vi "CheckModuleID.vi"(8 "Error In":errorcluster, 11 "Modle ID Array In":string[][](array[string])=[["12E", "4E"]]) -> (0 "Error Out":errorcluster, 3 "Modle ID ArrayOut":string[][](array[string])=[["12E", "4E"]])   [LabVIEW 2018, in "SensorPlugins.lvlib" / "RoomAlert.lvclass"]
doc: "Checks the Module ID to ensure we are only sending commands to the 4E and 12E since those are the only currently supported devices."
uses:
  RoomAlert.lvclass
  <vilib>/Utility/error.llb/Error Cluster From Error Code.vi
  <vilib>/ErrorRing/Error Ring.xnode
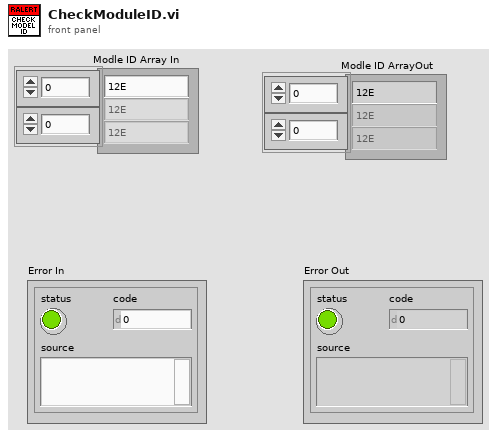
[diagram p1: front panel]
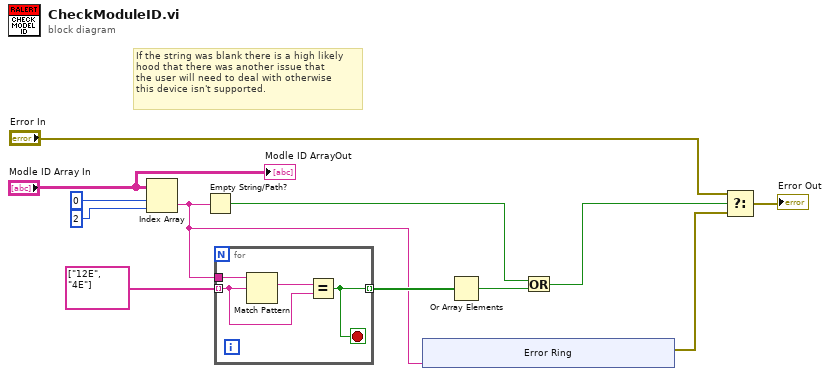
[diagram p0: block diagram]
diagram:
  # "If the string was blank there is a high likely \nhood that there was another issue that\nthe user will need to deal with otherwise\nthis device isn't supported."
  n1 = Index Array(array="Modle ID Array In", index (row)=0, index (col)=2 ("disabled index (col)")) -> (element=w4:string)
  n2 = Empty String/Path?(string/path=w4) -> (empty?=w7:bool)
  n3 = for {
    tunnel: w4 -> [w16]
    tunnel: string[] ["12E", "4E"] -> [w15] mode=indexing
    tunnel: [w13] -> w9 mode=indexing
    stop <- w13 stop-if-true
    n4 = Match Pattern(string=w16, regular expression=w15) -> (match substring=w14:string)  [unwired: 1 in, 3 out]
    n5 = Equal?(x=w14, y=w15) -> (x = y?=w13:bool)
  }
  n6 = xnode "Error Ring"("parameter 0"=w4) -> ("error out"=w5:errorcluster)
  n7 = Or Array Elements(Boolean array=w9) -> (logical OR=w8:bool)
  n8 = Or(x=w7, y=w8) -> (x .or. y?=w6:bool)
  n9 = Select(t="Error In", s=w6, f=w5) -> (s? t:f=→"Error Out":errorcluster)
  "Modle ID ArrayOut" <- "Modle ID Array In"
